vi "Abort Test.vi"(8 "error in (no error)":errorcluster, 11 "Generic Execution Adapter in":refnum<class "Generic Execution Adapter.lvclass">) -> (0 "error out":errorcluster, 2 "Abort Supported":bool, 3 "Generic Execution Adapter out":refnum<class "Generic Execution Adapter.lvclass">)   [LabVIEW 2026, in "Generic Execution Adapter.lvclass"]
uses:
  Generic Execution Adapter.lvclass
  Generic Execution Adapter.lvclass/Generic Execution Adapter.ctl
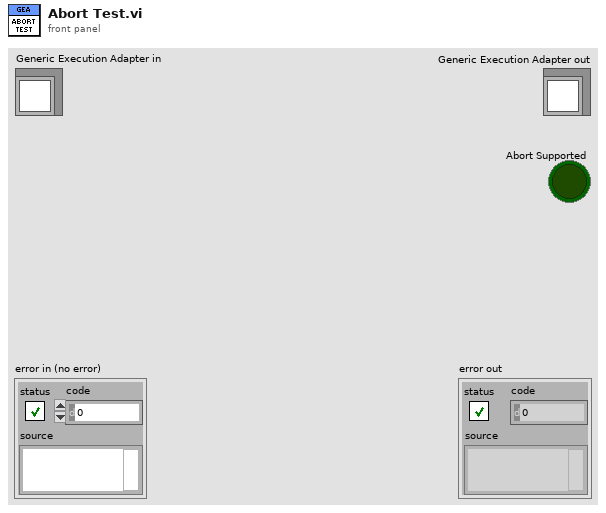
[diagram p1: front panel]
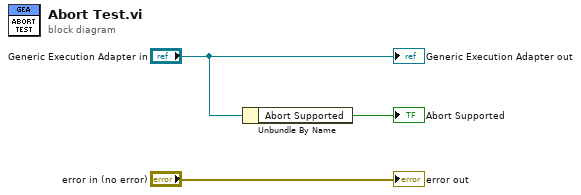
[diagram p0: block diagram]
diagram:
  n1 = Unbundle By Name("Generic Execution Adapter in") -> ("Abort Supported"=→"Abort Supported":bool)
  "error out" <- "error in (no error)"
  "Generic Execution Adapter out" <- "Generic Execution Adapter in"
